vi "Collapse Animation Done Callback.vi"(11 "Owner":refnum<class>) -> ()   [LabVIEW 2020, in "PicoG-Processor.lvlib" / "GVIWebProcessorApp.lvclass"]
uses:
  GVIWebProcessorApp.lvclass
  GVIWebProcessorApp.lvclass/GVIWebProcessorApp.ctl
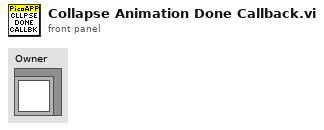
[diagram p1: front panel]
types:
  T1 = typedef "PicoG-Processor.lvlib/GVIWebProcessorApp.lvclass/Ref Data.ctl" = cluster{"hWnd":i32, "UI Refs":T2, "Collapsed":bool, "Async Anim Ref":refnum<vi>, "Expanded Bounds":T3, "Expanding":bool, "Collapsing":bool}
  T2 = typedef "PicoG-Processor.lvlib/GVIWebProcessorApp.lvclass/UI Refs.ctl" = cluster{"Main Window":refnum<vi>, "List Panel":refnum<vi>, "H Splitter":refnum<vi>, "V Splitter":refnum<vi>, "Open Project":refnum<vi>, "Project Name":refnum<vi>}
  T3 = typedef "LVRectTypeDef.ctl" = cluster{"Left":i16, "Top":i16, "Right":i16, "Bottom":i16}
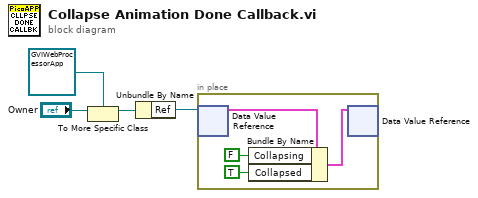
[diagram p0: block diagram]
diagram:
  n1 = To More Specific Class(target class=refnum<class "GVIWebProcessorApp.lvclass"> refnum ("PicoG-Processor:GVIWebProcessorApp.lvclass"), reference="Owner") -> (specific class reference=w1:refnum<class "GVIWebProcessorApp.lvclass">)  [unwired: 1 in, 1 out]
  n2 = Unbundle By Name(w1) -> ("Ref"=w2:refnum<data-value>)
  n3 = in-place {
    n4 = in-place-dvr #1(w2) -> (w8:T1)  [unwired: 1 out]
    n5 = Bundle By Name(cluster=w8, "Collapsing"=FALSE, "Collapsed"=TRUE) -> (w7:T1)
    n6 = in-place-dvr #1(w7) -> ()  [unwired: 2 out]
  }
